vi "Write.vi"(6 "Append Index":i32, 8 "error in (no error)":errorcluster, 9 "Notes":string, 10 "Data (Dictionary)":T1[](array[typedef]), 11 "Data.DAT in":refnum<class "Data.DAT.lvclass">) -> (0 "error out":errorcluster, 3 "Data.DAT out":refnum<class "Data.DAT.lvclass">, 5 "Path out":path)   [LabVIEW 2016, in "Data.DAT.lvclass"]
uses:
  Data.DAT.lvclass
  C:/user/patrick/git/LV-to-ITX/src/Data/Data.lvclass
  Data/Typedefs/Dictionary--cluster.ctl
  Data/Data.lvclass/Data.ctl
  Write DAT (2D).vi
  Data/Data.lvclass
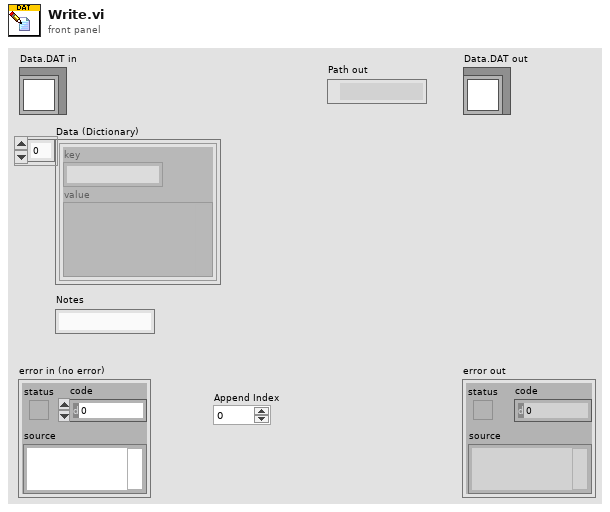
[diagram p1: front panel]
types:
  T1 = typedef "Data.lvclass/Dictionary--cluster.ctl" = cluster{"key":string, "value":variant}
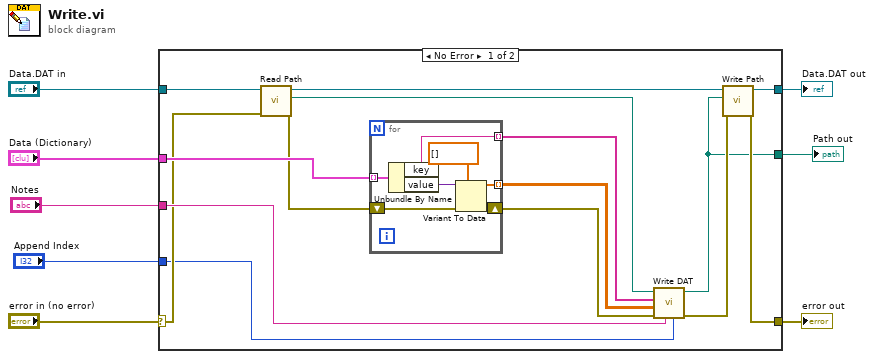
[diagram p0: block diagram]
diagram:
  n1 = case shown="No Error" "error in (no error)" {
    selector: "error in (no error)" -> [w12 w32]
    tunnel: [w21 w32] -> w7
    tunnel: "Data.DAT in" -> [w11 w31]
    tunnel: [w23 w31] -> w5
    tunnel: "Data (Dictionary)" -> [w16 _]
    tunnel: "Notes" -> [w13 _]
    tunnel: [w10 _] -> w2
    tunnel: "Append Index" -> [w9 _]
    frame No Error {
      n2 = call "Read Path.vi"("error in (no error)"=w12, "Data Save"=w11) -> ("error out"=w14:errorcluster, "Path"=w15:path, "Data Save out"=w18:refnum<class "Data.DAT.lvclass">)  [unwired: 7 in]
      n3 = for {
        tunnel: w16 -> [w30] mode=indexing
        tunnel: [w25] -> w19 mode=indexing
        tunnel: [w24] -> w17 mode=indexing
        shift-right: [w27] -> w20
        shift-left: w14 -> [w28]
        n4 = Unbundle By Name(w30) -> ("key"=w25:string, "value"=w29:variant)
        n5 = Variant To Data(error in=w28, type=dbl[] [] ("Data"), Variant=w29) -> (data=w24:dbl[], error out=w27:errorcluster)
      }
      n6 = call-poly "Write DAT.vi"("Append (0=F)"=w9, "Comments"=w13, "error in"=w20, "Data"=w17, "Headers"=w19, "path"=w15) -> ("error out"=w22:errorcluster, "new file path"=w10:path)  [unwired: 4 in]
      n7 = call "Write Path.vi"("error in (no error)"=w22, "Path"=w10, "Data Save"=w18) -> ("error out"=w21:errorcluster, "Data Save out"=w23:refnum<class "Data.DAT.lvclass">)  [unwired: 7 in]
    }
    frame Error {
    }
  }
  "error out" <- w7
  "Data.DAT out" <- w5
  "Path out" <- w2
